vi "n set fly rot.vi"(8 "error in (no error)":errorcluster, 10 "resolution":dbl, 11 "n":u16) -> (0 "error out":errorcluster)   [LabVIEW 2015, in "SCANalone4x64.lvlib"]
doc: "__declspec(dllimport) void __stdcall n_set_fly_rot(unsigned short n, double resolution);"
uses:
  <userlib>/SCANalone4x64/SCANalone4x64.lvlib
  <userlib>/SCANalone4x64/SCANalone4x64.dll
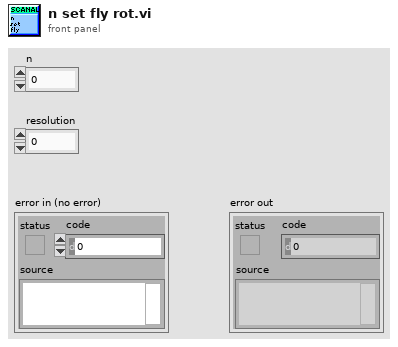
[diagram p1: front panel]
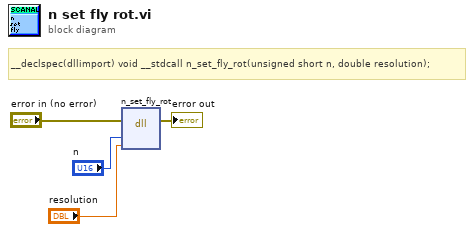
[diagram p0: block diagram]
diagram:
  # "__declspec(dllimport) void __stdcall n_set_fly_rot(unsigned short n, double resolution);"
  n1 = dll-call lib="C:/Program Files/National Instruments/LabVIEW 2015/user.lib/SCANalone4x64/SCANalone4x64.*" fn="n_set_fly_rot"(error in="error in (no error)", "n"="n", "resolution"="resolution") -> (error out=→"error out":errorcluster)  [unwired: 5 in, 1 out]
